vi "Get Audio Data.vi"(8 "error in (no error)":errorcluster, 11 "Kinect Session in":refnum<class "Kinect Session.lvclass">) -> (0 "error out":errorcluster, 1 "SoundSourceAngleConfidence":dbl, 2 "SoundSourceAngle":dbl, 3 "Kinect Session out":refnum<class "Kinect Session.lvclass">, 4 "BeamAngle":dbl)   [LabVIEW 2014, in "Kinect Library.lvlib"]
doc: "This function returns the post-processed attempt to find the users location based on the sound they produce. The angle is 0 when the user is directly in front of the camera and is in degrees."
uses:
  Kinect Library.lvlib
  Kinect Session Class/Kinect Session.lvclass
  Microsoft.Kinect
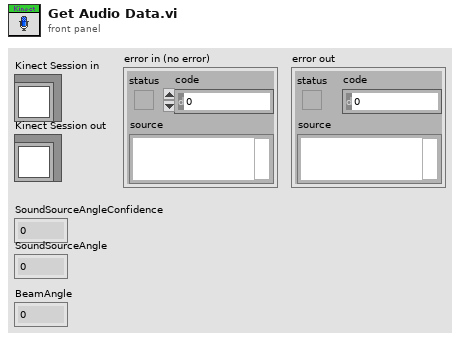
[diagram p1: front panel]
types:
  T1 = cluster{"status":bool, "code":bool, "source":bool}
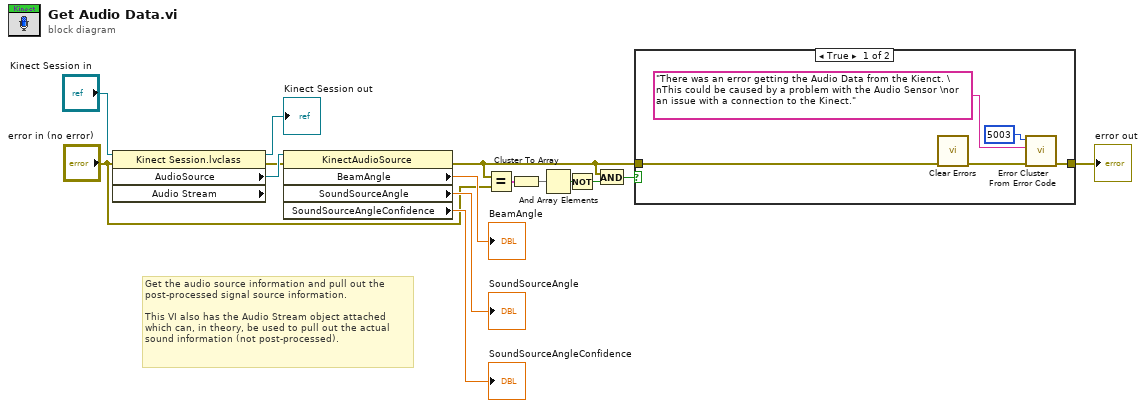
[diagram p0: block diagram]
diagram:
  # "Get the audio source information and pull out the\npost-processed signal source information.\n\nThis VI also has the Audio Stream object attached\nwhich can, in theory, be used to pull out the actual\nsound information (not post-processed)."
  n1 = property class="Kinect Session.lvclass" props=["AudioSource", "Audio Stream"](reference="Kinect Session in", error in="error in (no error)") -> (reference out=→"Kinect Session out":refnum<class "Kinect Session.lvclass">, error out=w14:errorcluster, "AudioSource"=w15:refnum<k24>)  [unwired: 1 out]
  n2 = property class="KinectAudioSource"(reference=w15, error in=w14) -> (error out=w4:errorcluster, "BeamAngle"=→"BeamAngle":dbl, "SoundSourceAngle"=→"SoundSourceAngle":dbl, "SoundSourceAngleConfidence"=→"SoundSourceAngleConfidence":dbl)  [unwired: 1 out]
  n3 = Equal?(x=w4, y="error in (no error)") -> (x = y?=w8:T1)
  n4 = Cluster To Array(cluster=w8) -> (array=w7:bool[])
  n5 = And Array Elements(Boolean array=w7) -> (logical AND=w1:bool)
  n6 = Not(x=w1) -> (.not. x?=w6:bool)
  n7 = And(x=w4, y=w6) -> (x .and. y?=w3:bool)
  n8 = case shown="True" w3 {
    tunnel: [w16 w21] -> w2
    tunnel: w4 -> [w18 w21]
    frame True {
      n9 = call <vilib>:"Clear Errors.vi"("error in (no error)"=w18) -> ("error out"=w17:errorcluster)  [unwired: 5 in, 1 out]
      n10 = call <vilib>:"Error Cluster From Error Code.vi"("error in (no error)"=w17, "error message (\"\")"="There was an error getting the Audio Data from the Kienct. \nThis could be caused by a problem with the Audio Sensor \nor an issue with a connection to the Kinect." ("error message (\"\")"), "error code (0)"=5003) -> ("error out"=w16:errorcluster)  [unwired: 6 in]
    }
    frame False {
    }
  }
  "error out" <- w2
